vi "Data Array.vi"(8 "error in (no error)":errorcluster, 11 "Node Ptr":T1 format="%.0x") -> (0 "error out":errorcluster)   [LabVIEW 2019, in "OPC UA Client Addon System Explorer.lvlib"]
uses:
  OPC UA Client Addon System Explorer.lvlib
  <vilib>/NI VeriStand/Custom Device API/Custom Device API.lvlib
  Addon Shared/Constants.vi
  Addon Shared/OPC UA Client Addon Shared.lvlib
  <vilib>/NI VeriStand/Custom Device API/Get Item Property (U32).vi
  <vilib>/NI VeriStand/Custom Device API/Get Item Property (String).vi
  <vilib>/NI VeriStand/Custom Device API/Custom Device Item Ref.ctl
panel:
  out "Tag Path":string
  out "DataType":u32(ring)=1 items=["Boolean"=1, "SByte"=2, "Byte"=3, "Int16"=4, "UInt16"=5, "Int32"=6, "UInt32"=7, "Int64"=8, "UInt64"=9, "Float"=10, "Double"=11, "String"=12, "DateTime"=13, "ByteString"=15, "Array of Boolean"=101, "Array of SByte"=102, "Array of Byte"=103, "Array of Int16"=104, "Array of UInt16"=105, "Array of Int32"=106, "Array of UInt32"=107, "Array of Int64"=108, "Array of UInt64"=109, "Array of Float"=110, "Array of Double"=111, "Array of String"=112, "Array of DateTime"=113, "Array of ByteString"=115]
  out "Array Size":i32
  in  "SHDocVw.IWebBrowser":refnum<k7>(container)
  in  "Header":cluster{"Section Name":string}={"Section Name"="Custom Device Item Settings"}
  in  "Description":string
  out "Name":string
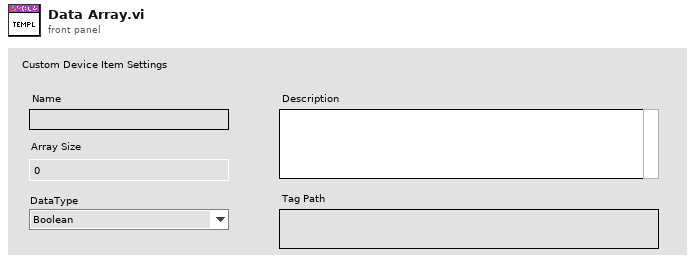
[diagram p1: front panel]
types:
  T1 = typedef "Custom Device API.lvlib/Custom Device Item Ref.ctl" = u64
  T2 = typedef "Custom Device API.lvlib/Custom Device Item Info.ctl" = cluster{"Name":string, "Is Channel":bool, "GUID":string, "Is Waveform":bool}
  T3 = typedef "Custom Device API.lvlib/Custom Device Commands.ctl" = enum16{"Default", "Item renamed", "Shutdown", "Dynamic button pressed"}
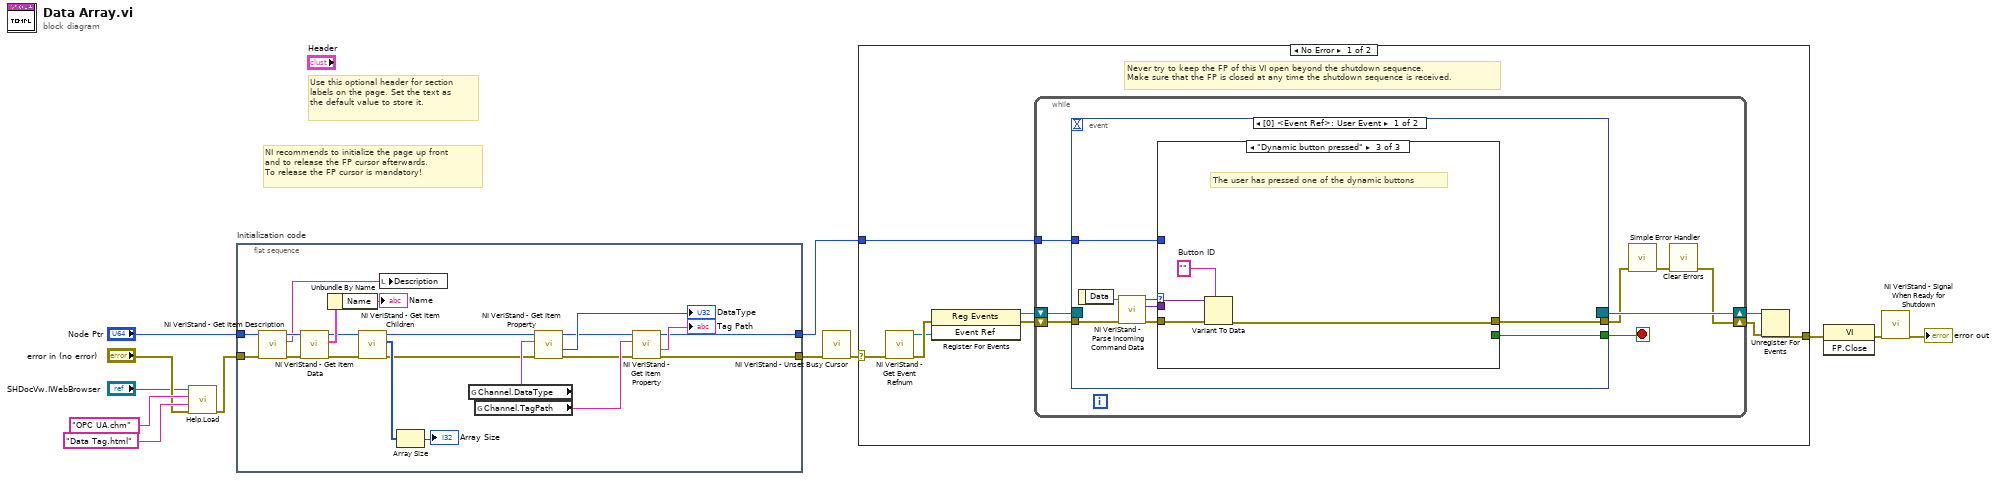
[diagram p0: block diagram]
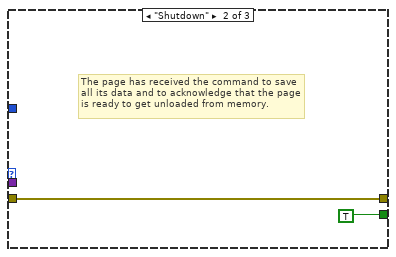
[diagram p3: hidden frame]
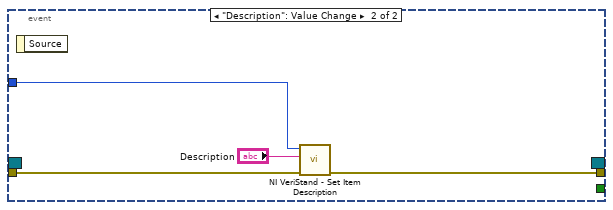
[diagram p4: hidden frame]
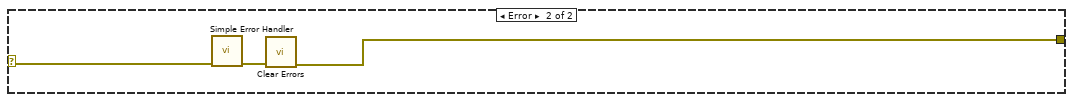
[diagram p5: hidden frame]
diagram:
  # "Use this optional header for section labels on the page. Set the text as the default value to store it."
  # "NI recommends to initialize the page up front\nand to release the FP cursor afterwards.\nTo release the FP cursor is mandatory!"
  n1 = call "Help.Load.vi"("error in (no error)"="error in (no error)", "HTML File"="Data Tag.html" ("Main CHM File"), "Main CHM File"="OPC UA.chm", "SHDocVw.IWebBrowser2"="SHDocVw.IWebBrowser") -> ("error out"=w2:errorcluster)  [unwired: 7 in]
  n2 = flat-sequence "Initialization code" {
    tunnel: w2 -> [w32]
    tunnel: "Node Ptr" -> [w31]
    tunnel: [w15] -> w8
    tunnel: [w13] -> w6
    frame #0 {
      n3 = call <vilib>:"NI VeriStand - Get Item Description.vi"("error in (no error)"=w32, "Item Ref in"=w31) -> ("error out"=w29:errorcluster, "Description"=w30:string, "Item Ref out"=w33:T1)  [unwired: 7 out]
      n4 = call <vilib>:"NI VeriStand - Get Item Data.vi"("error in (no error)"=w29, "Item Ref in"=w33) -> ("error out"=w26:errorcluster, "Item Info"=w28:T2, "Item Ref out"=w25:T1)  [unwired: 7 out]
      n5 = Unbundle By Name(w28) -> ("Name"=→"Name":string)
      n6 = call <vilib>:"NI VeriStand - Get Item Children.vi"("error in (no error)"=w26, "Item Ref in"=w25) -> ("error out"=w16:errorcluster, "Child Refs"=w24:T1[], "Item Ref out"=w14:T1)  [unwired: 6 in, 1 out]
      n7 = local write "Description"(w30) -> ()
      n8 = Array Size(array=w24) -> (size(s)=→"Array Size":i32)
      n9 = global read "Constants.vi" "Channel.DataType"() -> (w19:string)
      n10 = global read "Constants.vi" "Channel.TagPath"() -> (w20:string)
      n11 = call-poly <vilib>:"NI VeriStand - Get Item Property.vi"("error in (no error)"=w16, "Property Name"=w19, "Item Ref in"=w14) -> ("error out"=w18:errorcluster, "Value"=→"DataType":u32, "Item Ref out"=w17:T1)  [unwired: 5 in, 1 out]
      n12 = call-poly <vilib>:"NI VeriStand - Get Item Property.vi"("error in (no error)"=w18, "Property Name"=w20, "Item Ref in"=w17) -> ("error out"=w15:errorcluster, "Value"=→"Tag Path":string, "Item Ref out"=w13:T1)  [unwired: 5 in, 1 out]
    }
  }
  n13 = call <vilib>:"NI VeriStand - Unset Busy Cursor.vi"("error in (no error)"=w8) -> ("error out"=w7:errorcluster)  [unwired: 10 out]
  n14 = case shown="No Error" w7 {
    selector: w7 -> [w34 w72]
    tunnel: [w39 w70] -> w12
    tunnel: w6 -> [w35 _]
    frame No Error {
      # "Never try to keep the FP of this VI open beyond the shutdown sequence.\nMake sure that the FP is closed at any time the shutdown sequence is received."
      n15 = call <vilib>:"NI VeriStand - Get Event Refnum.vi"("error in (no error)"=w34) -> ("error out"=w42:errorcluster, "Event Ref"=w38:refnum<user-event>)  [unwired: 9 out]
      n16 = register-events(error in=w42, w38) -> (reference out=w36:refnum<event-registration>, error out=w37:errorcluster)  [unwired: 1 in]
      n17 = while {
        tunnel: w35 -> [w46]
        shift-right: [w43] -> w40
        shift-left: w37 -> [w49]
        shift-right: [w50] -> w41
        shift-left: w36 -> [w48]
        stop <- w47 stop-if-true
        n18 = event shown="[0] <Event Ref>: User Event" {
          selector: w48 -> [_ _]
          dyn-events: [_ _] -> w50
          timeout: _ -> [_ _]
          tunnel: w49 -> [w58 w68]
          tunnel: [w54 _] -> w47
          tunnel: [w53 w67] -> w45
          tunnel: w46 -> [w52 w69]
          event User Event {
            n19 = event-data() -> ("Data"=w57:string)  [unwired: 1 out]
            n20 = call <vilib>:"NI VeriStand - Parse Incoming Command Data.vi"("error in (no error)"=w58, "Incoming data"=w57) -> ("error out"=w56:errorcluster, "Outgoing data"=w51:variant, "Action"=w55:T3)  [unwired: 7 out]
            n21 = case shown="\"Dynamic button pressed\"" w55 {
              tunnel: w56 -> [w59 w60 w65]
              tunnel: [_ TRUE _] -> w54
              tunnel: [w59 w60 w62] -> w53
              tunnel: w52 -> [_ _ _]
              tunnel: w51 -> [_ _ w64]
              frame "Default", Default {
              }
              frame "Shutdown" {
                # "The page has received the command to save all its data and to acknowledge that the page is ready to get unloaded from memory."
              }
              frame "Dynamic button pressed" {
                w63 = ""  # Button ID
                # "The user has pressed one of the dynamic buttons"
                n22 = Variant To Data(error in=w65, type=w63, Variant=w64) -> (error out=w62:errorcluster)  [unwired: 1 out]
              }
            }
          }
          event "Description": Value Change {
            n23 = event-data() -> ()  [unwired: 2 out]
            n24 = call <vilib>:"NI VeriStand - Set Item Description.vi"("error in (no error)"=w68, "Description"="Description", "Item Ref in"=w69) -> ("error out"=w67:errorcluster)  [unwired: 8 out]
          }
        }
        n25 = call <vilib>:"Simple Error Handler.vi"("error in (no error)"=w45) -> ("error out"=w44:errorcluster)  [unwired: 1 in, 7 out]
        n26 = call <vilib>:"Clear Errors.vi"("error in (no error)"=w44) -> ("error out"=w43:errorcluster)  [unwired: 1 in, 5 out]
      }
      n27 = Unregister For Events(event registration refnum=w41, error in=w40) -> (error out=w39:errorcluster)
    }
    frame Error {
      n28 = call <vilib>:"Simple Error Handler.vi"("error in (no error)"=w72) -> ("error out"=w71:errorcluster)  [unwired: 1 in, 7 out]
      n29 = call <vilib>:"Clear Errors.vi"("error in (no error)"=w71) -> ("error out"=w70:errorcluster)  [unwired: 1 in, 5 out]
    }
  }
  n30 = invoke class="VI" method="FP.Close"(error in=w12) -> (error out=w11:errorcluster)  [unwired: 2 in, 2 out]
  n31 = call <vilib>:"NI VeriStand - Signal When Ready for Shutdown.vi"("error in (no error)"=w11) -> ("error out"=→"error out":errorcluster)  [unwired: 10 out]
